vi "StahlPS_USB.set device state.vi"(0 "i ref in":refnum<vi>, 1 "deviceState":T1 items=["ERROR"=-1, "OK"=0, "NOT_OK"=1], 2 "implicit":bool, 3 "ms timeout (10000)":i32=10000, 4 "device error":errorcluster, 5 "error in (no error)":errorcluster, 7 "mayResetError (FALSE)":bool) -> (14 "i ref out":refnum<vi>, 17 "timed out":bool, 19 "error out":errorcluster)   [LabVIEW 2014, in "StahlPS_USB.lvlib"]
doc: "This is an override method to take care of class specific stuff in the \"calculation\" of the device state.\n\nSets the state of a device. There are three device states\n\n0 : OK\n>0: NOT_OK\n<0: ERROR \n\nIn case the device state is set \"implicitely\", the severity of the \"device error\" is analyzed. In case of \"fatal\" or \"error\", the device state is set to \"ERROR\". In case of \"warning\", the device state is set to \"NOT_OK\". In all other cases, the device state is set to \"OK\".\n\nPer default, the device state can not be changed in case of \"ERROR\". If one wants to reset the device state one has to call THIS method with the option mayResetError set to TRUE."
uses:
  StahlPS_USB.lvlib
  CSCore/CSApplicationBaseClasses/DeviceBase/DeviceBase.deviceState.ctl
  CSCore/CSApplicationBaseClasses/PSChannelBase/PSChannelBase.statusType.ctl
  CSCore/CSApplicationBaseClasses/PSChannelBase/PSChannelBase.serviceType.ctl
  CSCore/CSApplicationBaseClasses/PSChannelBase/PSChannelBase.directionType.ctl
  CSCore/CSApplicationBaseClasses/DeviceBase/DeviceBase.lvlib
  CSCore/CSApplicationBaseClasses/PSChannelBase/PSChannelBase.lvlib
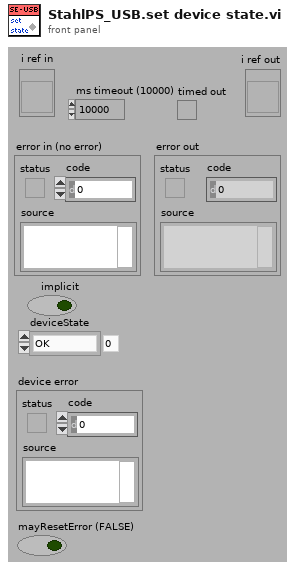
[diagram p1: front panel]
types:
  T1 = typedef "DeviceBase.lvlib/DeviceBase.deviceState.ctl" = i16
  T2 = typedef "PSChannelBase.lvlib/PSChannelBase.directionType.ctl" = enum16{"unknown", "update actual value", "update nominal value", "update both"}
  T3 = typedef "PSChannelBase.lvlib/PSChannelBase.serviceType.ctl" = enum16{"onOff", "voltage", "current", "tripCurrent", "rampUpSpeed", "rampDownSpeed", "status"}
  T4 = typedef "PSChannelBase.lvlib/PSChannelBase.statusType.ctl" = i32
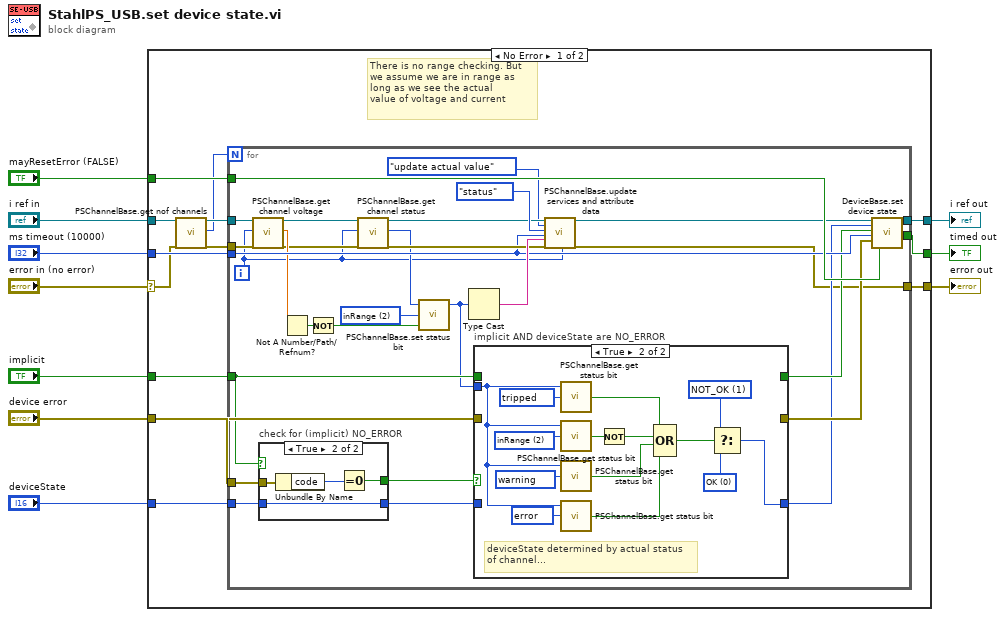
[diagram p0: block diagram]
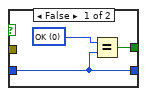
[diagram p3: hidden frame]
diagram:
  n1 = case shown="No Error" "error in (no error)" {
    selector: "error in (no error)" -> [w12 w78]
    tunnel: [w22 _] -> w10
    tunnel: [w16 w79] -> w9
    tunnel: "ms timeout (10000)" -> [w21 _]
    tunnel: "implicit" -> [w18 _]
    tunnel: "i ref in" -> [w15 w79]
    tunnel: "device error" -> [w19 _]
    tunnel: "deviceState" -> [w20 _]
    tunnel: [w17 w78] -> w2
    tunnel: "mayResetError (FALSE)" -> [w23 _]
    frame No Error {
      # "There is no range checking. But\nwe assume we are in range as\nlong as we see the actual\nvalue of voltage and current"
      n2 = call "PSChannelBase.get nof channels.vi"("i ref in"=w15, "error in (no error)"=w12) -> ("i ref out"=w14:refnum<vi>, "NofChannels"=w11:i32, "error out"=w13:errorcluster)  [unwired: 15 in]
      n3 = for {
        N: w11 -> [_]
        tunnel: w23 -> [w53]
        tunnel: [w52] -> w22
        tunnel: w21 -> [w45]
        tunnel: w20 -> [w44]
        tunnel: w19 -> [w42]
        tunnel: w18 -> [w39]
        tunnel: [w34] -> w17
        tunnel: [w33] -> w16
        tunnel: w14 -> [w26]
        tunnel: w13 -> [w25]
        i -> [w24]
        w47 = T4 2 items=["onOff"=1, "inRange"=2, "rampingUp"=4, "rampingDown"=8, "currentRegulated"=16, "voltageRegulated"=32, "reserved1"=64, "reserved2"=128, "reserved3"=256, "reserved4"=512, "reserved5"=1024, "reserved6"=2048, "reserved7"=4096, "reserved8"=8192, "reserved9"=16384, "reserved10"=32768, "reserved11"=65536, "user1"=131072, "user2"=262144, "user3"=524288, "user4"=1048576, "user5"=2097152, "user6"=4194304, "user7"=8388608, "user8"=16777216, "user9"=33554432, "user10"=67108864, "user11"=134217728, "tripped"=268435456, "warning"=536870912, "error"=1073741824] ("statusBit")
        n4 = call "PSChannelBase.get channel voltage.vi"("i ref in"=w26, "channelIndx"=w24, "error in (no error)"=w25) -> ("i ref out"=w28:refnum<vi>, "voltage"=w31:dbl, "error out"=w27:errorcluster)  [unwired: 14 in]
        n5 = case "check for (implicit) NO_ERROR" shown="True" w39 {
          tunnel: w42 -> [_ w77]
          tunnel: [w72 w75] -> w43
          tunnel: w44 -> [w71 w74]
          tunnel: [w71 w74] -> w41
          frame False {
            w73 = T1 0 items=["ERROR"=-1, "OK"=0, "NOT_OK"=1] ("x")
            n6 = Equal?(x=w73, y=w71) -> (x = y?=w72:bool)
          }
          frame True {
            n7 = Unbundle By Name(w77) -> ("code"=w76:i32)
            n8 = Equal To 0?(x=w76) -> (x = 0?=w75:bool)
          }
        }
        n9 = Not A Number/Path/Refnum?(number/path/refnum=w31) -> (NaN/Path/Refnum?=w30:bool)
        n10 = Not(x=w30) -> (.not. x?=w29:bool)
        n11 = call "PSChannelBase.get channel status.vi"("i ref in"=w28, "channelIndex"=w24, "error in (no error)"=w27) -> ("i ref out"=w48:refnum<vi>, "status"=w36:i32, "error out"=w50:errorcluster)  [unwired: 14 in]
        n12 = call "PSChannelBase.set status bit.vi"("set"=w29, "statusBit"=w47, "status"=w36) -> ("status out"=w32:T4)  [unwired: 2 in]
        n13 = Type Cast(x=w32) -> (*(type *) &x=w51:string)  [unwired: 1 in]
        n14 = case "implicit AND deviceState are NO_ERROR" shown="True" w43 {
          tunnel: w42 -> [w55 _]
          tunnel: w41 -> [w56 _]
          tunnel: [w56 w57] -> w37
          tunnel: [w55 _] -> w40
          tunnel: w39 -> [w54 _]
          tunnel: [w54 _] -> w38
          tunnel: w32 -> [_ w67]
          frame False {
          }
          frame True {
            w58 = T1 1 items=["ERROR"=-1, "OK"=0, "NOT_OK"=1] ("t")
            w59 = T1 0 items=["ERROR"=-1, "OK"=0, "NOT_OK"=1] ("deviceState")
            w66 = T4 1073741824 items=["onOff"=1, "inRange"=2, "rampingUp"=4, "rampingDown"=8, "currentRegulated"=16, "voltageRegulated"=32, "reserved1"=64, "reserved2"=128, "reserved3"=256, "reserved4"=512, "reserved5"=1024, "reserved6"=2048, "reserved7"=4096, "reserved8"=8192, "reserved9"=16384, "reserved10"=32768, "reserved11"=65536, "user1"=131072, "user2"=262144, "user3"=524288, "user4"=1048576, "user5"=2097152, "user6"=4194304, "user7"=8388608, "user8"=16777216, "user9"=33554432, "user10"=67108864, "user11"=134217728, "tripped"=268435456, "warning"=536870912, "error"=1073741824] ("statusBit")
            w68 = T4 536870912 items=["onOff"=1, "inRange"=2, "rampingUp"=4, "rampingDown"=8, "currentRegulated"=16, "voltageRegulated"=32, "reserved1"=64, "reserved2"=128, "reserved3"=256, "reserved4"=512, "reserved5"=1024, "reserved6"=2048, "reserved7"=4096, "reserved8"=8192, "reserved9"=16384, "reserved10"=32768, "reserved11"=65536, "user1"=131072, "user2"=262144, "user3"=524288, "user4"=1048576, "user5"=2097152, "user6"=4194304, "user7"=8388608, "user8"=16777216, "user9"=33554432, "user10"=67108864, "user11"=134217728, "tripped"=268435456, "warning"=536870912, "error"=1073741824] ("statusBit")
            w69 = T4 2 items=["onOff"=1, "inRange"=2, "rampingUp"=4, "rampingDown"=8, "currentRegulated"=16, "voltageRegulated"=32, "reserved1"=64, "reserved2"=128, "reserved3"=256, "reserved4"=512, "reserved5"=1024, "reserved6"=2048, "reserved7"=4096, "reserved8"=8192, "reserved9"=16384, "reserved10"=32768, "reserved11"=65536, "user1"=131072, "user2"=262144, "user3"=524288, "user4"=1048576, "user5"=2097152, "user6"=4194304, "user7"=8388608, "user8"=16777216, "user9"=33554432, "user10"=67108864, "user11"=134217728, "tripped"=268435456, "warning"=536870912, "error"=1073741824] ("statusBit")
            w70 = T4 268435456 items=["onOff"=1, "inRange"=2, "rampingUp"=4, "rampingDown"=8, "currentRegulated"=16, "voltageRegulated"=32, "reserved1"=64, "reserved2"=128, "reserved3"=256, "reserved4"=512, "reserved5"=1024, "reserved6"=2048, "reserved7"=4096, "reserved8"=8192, "reserved9"=16384, "reserved10"=32768, "reserved11"=65536, "user1"=131072, "user2"=262144, "user3"=524288, "user4"=1048576, "user5"=2097152, "user6"=4194304, "user7"=8388608, "user8"=16777216, "user9"=33554432, "user10"=67108864, "user11"=134217728, "tripped"=268435456, "warning"=536870912, "error"=1073741824] ("statusBit")
            # "deviceState determined by actual status\nof channel..."
            n15 = call "PSChannelBase.get status bit.vi"("statusBit"=w70, "status"=w67) -> ("set"=w65:bool)  [unwired: 3 in]
            n16 = call "PSChannelBase.get status bit.vi"("statusBit"=w69, "status"=w67) -> ("set"=w62:bool)  [unwired: 3 in]
            n17 = call "PSChannelBase.get status bit.vi"("statusBit"=w68, "status"=w67) -> ("set"=w63:bool)  [unwired: 3 in]
            n18 = call "PSChannelBase.get status bit.vi"("statusBit"=w66, "status"=w67) -> ("set"=w64:bool)  [unwired: 3 in]
            n19 = Not(x=w62) -> (.not. x?=w61:bool)
            n20 = Compound Arithmetic op=OR(w65, w61, w63, w64) -> (w60:bool)
            n21 = Select(t=w58, s=w60, f=w59) -> (s? t:f=w57:T1)
          }
        }
        n22 = call "PSChannelBase.update services and attribute data.vi"("i ref in"=w48, "direction"=PSChannelBase.directionType."update actual value", "service"=PSChannelBase.serviceType."status", "ms timeout (10000)"=w45, "value"=w51, "error in (no error)"=w50, "channelNumber"=w24) -> ("i ref out"=w35:refnum<vi>, "error out"=w34:errorcluster)  [unwired: 10 in, 1 out]
        n23 = call "DeviceBase.set device state.vi"("i ref in"=w35, "deviceState"=w37, "implicit"=w38, "ms timeout (10000)"=w45, "device error"=w40, "mayResetError (FALSE)"=w53) -> ("i ref out"=w33:refnum<vi>, "timed out"=w52:bool)  [unwired: 11 in, 1 out]
      }
    }
    frame Error {
    }
  }
  "error out" <- w2
  "i ref out" <- w9
  "timed out" <- w10
